vi "TOPAZ.vi"(2 "stop":bool, 4 "wait":u32=250, 6 "Отправить команду":bool, 8 "Ослабление, дБ":ext format="%.2g", 9 "Длина волны, нм":enum16{"850", "1300", "1310", "1550"}(ring), 10 "Выбор команды:":T2(ring), 11 "COM-порт":refnum<visa-resource-name>="COM7") -> (3 "Ответ устройства:":string, 5 "прочитано":u32, 7 "отправлено":u32)   [LabVIEW 2018]
uses:
  <vilib>/Instr/_visa.llb/VISA Configure Serial Port (Instr).vi
panel:
  in  "Tab Control":T1(tab)
  # "Задание параметров:\nВбери команду!"
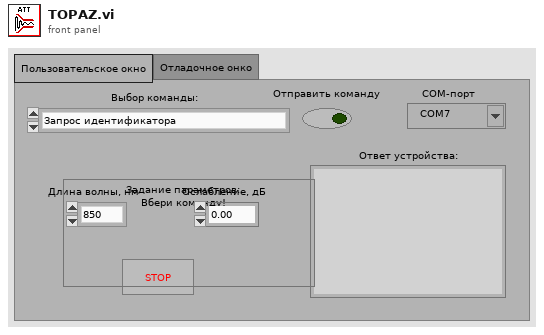
[diagram p1: front panel]
types:
  T1 = enum32{"Пользовательское окно", "Отладочное онко"}
  T2 = enum16{"Запрос идентификатора", "Запрос установленной длины волны, (нм)", "Запрос установленного ослабления, (дБ)", "Установка длины волны, (нм)", "Установка ослабления, (дБ)"}
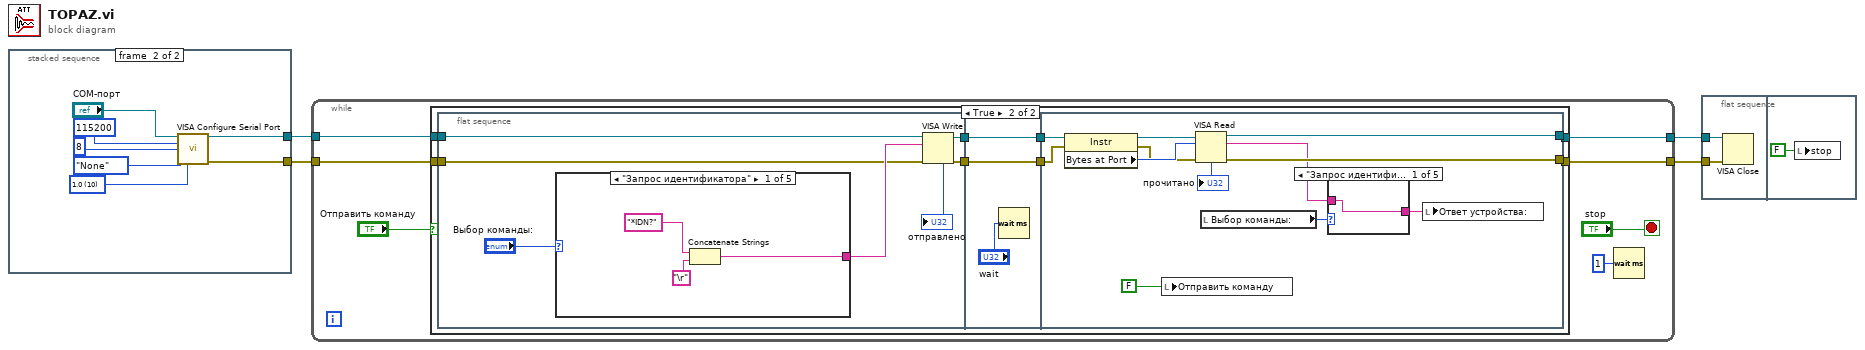
[diagram p0: block diagram]
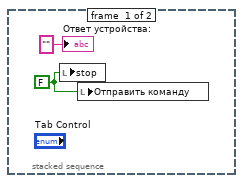
[diagram p2: hidden frame]
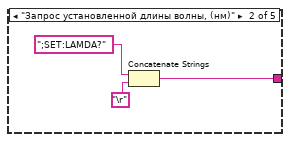
[diagram p4: hidden frame]
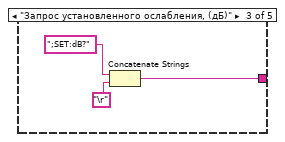
[diagram p5: hidden frame]
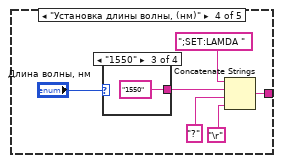
[diagram p6: hidden frame]
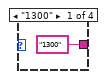
[diagram p7: hidden frame]
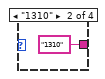
[diagram p8: hidden frame]
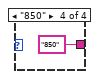
[diagram p9: hidden frame]
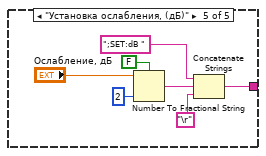
[diagram p10: hidden frame]
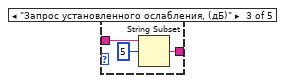
[diagram p12: hidden frame]
diagram:
  n1 = stacked-sequence {
    tunnel: [_ w8] -> w2
    tunnel: [_ w7] -> w1
    frame #0 {
      w5 = FALSE ("Текущее\nослабление? (дБ)")
      n2 = local write "stop"(w5) -> ()
      n3 = local write "Отправить команду"(w5) -> ()
      "Ответ устройства:" <- "" ("Ответ:")
    }
    frame #1 {
      w10 = u16 10 items=["1.0"=10, "1.5"=15, "2.0"=20] ("stop bits (10: 1 bit)")
      n4 = call-poly "VISA Configure Serial Port"("VISA resource name"="COM-порт", "baud rate (9600)"=u32 115200, "data bits (8)"=u16 8, "parity (0:none)"=enum16{"None", "Odd", "Even", "Mark", "Space"}."None", "stop bits (10: 1 bit)"=w10) -> ("VISA resource name out"=w8:refnum<visa-resource-name>, "error out"=w7:errorcluster)  [unwired: 9 in]
    }
  }
  n5 = while {
    tunnel: [w18] -> w4
    tunnel: [w17] -> w3
    tunnel: w2 -> [w16]
    tunnel: w1 -> [w15]
    stop <- "stop" stop-if-true
    n6 = case shown="True" "Отправить команду" {
      tunnel: [w22 w28] -> w18
      tunnel: [w21 w25] -> w17
      tunnel: w16 -> [w22 w24]
      tunnel: w15 -> [w21 w23]
      frame False {
      }
      frame True {
        n7 = flat-sequence {
          tunnel: [w37] -> w29
          tunnel: [w35] -> w26
          tunnel: w24 -> [w34]
          tunnel: w23 -> [w31]
          tunnel: [w66] -> w30
          tunnel: w29 -> [w66]
          tunnel: [w65] -> w27
          tunnel: w26 -> [w65]
          tunnel: w30 -> [w76]
          tunnel: [w72] -> w28
          tunnel: w27 -> [w74]
          tunnel: [w71] -> w25
          frame #0 {
            n8 = case shown="\"Запрос идентификатора\"" "Выбор команды:" {
              tunnel: [w38 w41 w44 w47 w57] -> w32
              frame "Запрос идентификатора" {
                n9 = Concatenate Strings("*IDN?", "\r") -> (w38:string)
              }
              frame "Запрос установленной длины волны, (нм)" {
                n10 = Concatenate Strings(";SET:LAMDA?", "\r") -> (w41:string)
              }
              frame "Запрос установленного ослабления, (дБ)" {
                n11 = Concatenate Strings(";SET:dB?", "\r") -> (w44:string)
              }
              frame "Установка длины волны, (нм)" {
                n12 = case shown="\"1550\"" "Длина волны, нм" {
                  tunnel: ["1300" "1310" "1550" "850"] -> w48
                  frame "1300" {
                  }
                  frame "1310" {
                  }
                  frame "1550" {
                  }
                  frame "850" {
                  }
                }
                n13 = Concatenate Strings(";SET:LAMDA ", w48, "?" ("string"), "\r") -> (w47:string)
              }
              frame "Установка ослабления, (дБ)" {
                n14 = Number To Fractional String(use system decimal point (T)=FALSE, number="Ослабление, дБ", precision (6)=i16 2) -> (F-format string=w61:string)  [unwired: 1 in]
                n15 = Concatenate Strings(";SET:dB ", w61, "\r") -> (w57:string)
              }
            }
            n16 = VISA Write(VISA resource name=w34, write buffer=w32, error in (no error)=w31) -> (VISA resource name out=w37:refnum<visa-resource-name>, return count=→"отправлено":u32, error out=w35:errorcluster)
          }
          frame #1 {
            n17 = Wait (ms)(milliseconds to wait="wait") -> ()  [unwired: 1 out]
          }
          frame #2 {
            n18 = property class="Instr"(reference=w76, error in=w74) -> (reference out=w77:refnum<visa-resource-name>, error out=w70:errorcluster, "Bytes at Port"=w73:u32)
            n19 = local write "Отправить команду"(FALSE ("Текущее\nослабление? (дБ)")) -> ()
            n20 = VISA Read(VISA resource name=w77, byte count=w73, error in (no error)=w70) -> (VISA resource name out=w72:refnum<visa-resource-name>, read buffer=w68:string, return count=→"прочитано":u32, error out=w71:errorcluster)
            n21 = local read "Выбор команды:"() -> (w69:T2)
            n22 = case shown="\"Запрос идентификатора\", Default" w69 {
              tunnel: w68 -> [w79 w80 w82 w84 w85]
              tunnel: [w79 w80 w81 w84 w85] -> w67
              frame "Запрос идентификатора", Default {
              }
              frame "Запрос установленной длины волны, (нм)" {
              }
              frame "Запрос установленного ослабления, (дБ)" {
                n23 = String Subset(string=w82, offset (0)=5) -> (substring=w81:string)  [unwired: 1 in]
              }
              frame "Установка длины волны, (нм)" {
              }
              frame "Установка ослабления, (дБ)" {
              }
            }
            n24 = local write "Ответ устройства:"(w67) -> ()
          }
        }
      }
    }
    n25 = Wait (ms)(milliseconds to wait=u32 1) -> ()  [unwired: 1 out]
  }
  n26 = flat-sequence {
    tunnel: w4 -> [w87]
    tunnel: w3 -> [w86]
    frame #0 {
      n27 = VISA Close(VISA resource name=w87, error in (no error)=w86) -> ()  [unwired: 1 out]
    }
    frame #1 {
      n28 = local write "stop"(FALSE ("stop")) -> ()
    }
  }
